vi "CopyEndOfExistingFile.vi"(8 "error in (no error)":errorcluster, 11 "FileMerge in":refnum<class "FileMerge.lvclass">) -> (0 "error out":errorcluster, 3 "FileMerge out":refnum<class "FileMerge.lvclass">)   [LabVIEW 2018, in "FileMerge.lvclass"]
doc: "When test execution is complete, if there is any data remaining in the pre-existing merge data file, then copy it all over to the new file."
uses:
  FileMerge.lvclass
  FileMerge.lvclass/FileMerge.ctl
  ExistingFileMgr/ExistingFileMgr.lvclass
panel:
  out "i":i32
  out "Next File Index":i64 format="%.9p"
  out "starting File Index":i64 format="%.9p"
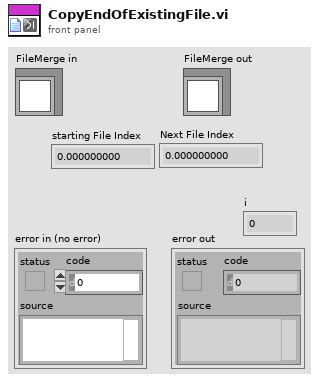
[diagram p1: front panel]
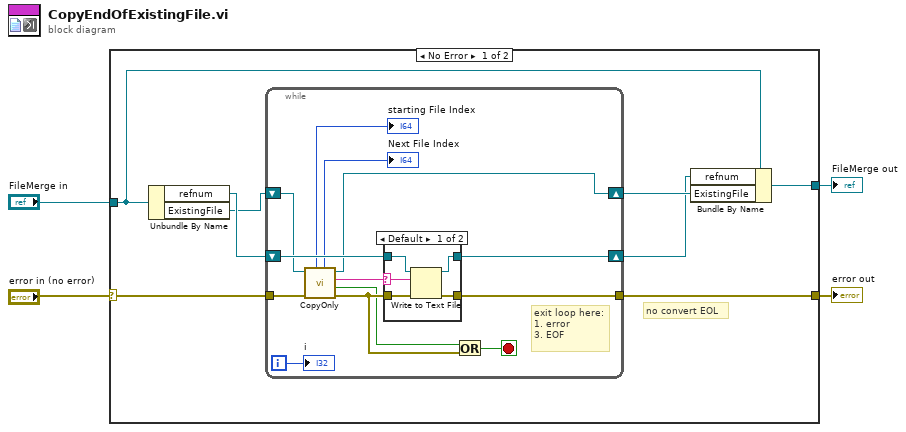
[diagram p0: block diagram]
diagram:
  n1 = case shown="No Error" "error in (no error)" {
    selector: "error in (no error)" -> [w7 w34]
    tunnel: [w5 w34] -> w3
    tunnel: [w9 w33] -> w1
    tunnel: "FileMerge in" -> [w10 w33]
    frame No Error {
      # "no convert EOL"
      n2 = Unbundle By Name(w10) -> ("refnum"=w12:refnum<file>, "ExistingFile"=w11:refnum<class "ExistingFileMgr.lvclass">)
      n3 = while {
        shift-right: [w22] -> w6
        shift-left: w12 -> [w25]
        shift-right: [w23] -> w8
        shift-left: w11 -> [w24]
        tunnel: w7 -> [w19]
        tunnel: [w18] -> w5
        i -> [w20]
        stop <- w16 stop-if-true
        # "exit loop here:\n1. error\n3. EOF"
        n4 = call "CopyOnly.vi"("error in (no error)"=w19, "ExistingFileMgr in"=w24) -> ("error out"=w17:errorcluster, "EOF=T"=w15:bool, "File Chunk to copy"=w21:string, "ExistingFileMgr out"=w23:refnum<class "ExistingFileMgr.lvclass">, "Next File Index"=→"Next File Index":i64, "starting File Index"=→"starting File Index":i64)  [unwired: 4 in]
        n5 = case shown="Default" w21 {
          selector: w21 -> [w26 _]
          tunnel: w25 -> [w30 w32]
          tunnel: [w29 w32] -> w22
          tunnel: [w28 w31] -> w18
          tunnel: w17 -> [w27 w31]
          frame Default {
            n6 = Write to Text File(file (use dialog)=w30, text=w26, error in=w27) -> (refnum out=w29:refnum<file>, error out=w28:errorcluster)  [unwired: 1 in, 1 out]
          }
          frame "" {
          }
        }
        n7 = Or(x=w15, y=w17) -> (x .or. y?=w16:bool)
        "i" <- w20
      }
      n8 = Bundle By Name(cluster=w10, "refnum"=w6, "ExistingFile"=w8) -> (w9:refnum<class "FileMerge.lvclass">)
    }
    frame Error {
    }
  }
  "error out" <- w3
  "FileMerge out" <- w1
